vi "Init Filtered System Mappings Tab.vi"(8 "error in (no error)":errorcluster, 11 "Loop Data in":T1) -> (0 "error out":errorcluster)   [LabVIEW 2016, in "System Mapping Tool.lvlib"]
uses:
  System Mapping Tool.lvlib
  TypeDefs/Loop Data.ctl
  TypeDefs/UI Refs.ctl
  NationalInstruments.VeriStand.SystemDefinitionAPI
  NationalInstruments.VeriStand.SystemStorageUI
  <vilib>/Utility/miscctls.llb/LVRowAndColumnTypeDef.ctl
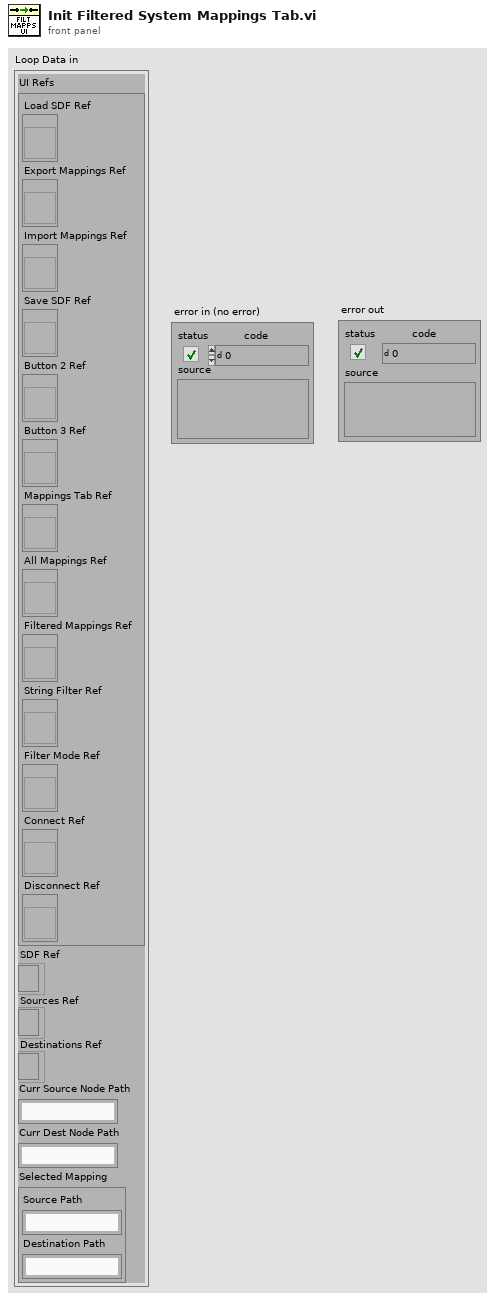
[diagram p1: front panel]
types:
  T1 = typedef "System Mapping Tool.lvlib/Loop Data.ctl" = cluster{"UI Refs":T2, "SDF Ref":refnum<k24>, "Sources Ref":refnum<k24>, "Destinations Ref":refnum<k24>, "Curr Source Node Path":string, "Curr Dest Node Path":string, "Selected Mapping":cluster{"Source Path":string, "Destination Path":string}}
  T2 = typedef "System Mapping Tool.lvlib/UI Refs.ctl" = cluster{"Load SDF Ref":refnum<vi>, "Export Mappings Ref":refnum<vi>, "Import Mappings Ref":refnum<vi>, "Save SDF Ref":refnum<vi>, "Button 2 Ref":refnum<vi>, "Button 3 Ref":refnum<vi>, "Mappings Tab Ref":refnum<vi>, "All Mappings Ref":refnum<vi>, "Filtered Mappings Ref":refnum<vi>, "String Filter Ref":refnum<vi>, "Filter Mode Ref":refnum<vi>, "Connect Ref":refnum<vi>, "Disconnect Ref":refnum<vi>}
  T3 = typedef "LVRowAndColumnTypeDef.ctl" = cluster{"Row":i32, "Column":i32}
  T4 = enum32{"All System Mappings", "Filtered Mappings by Node"}
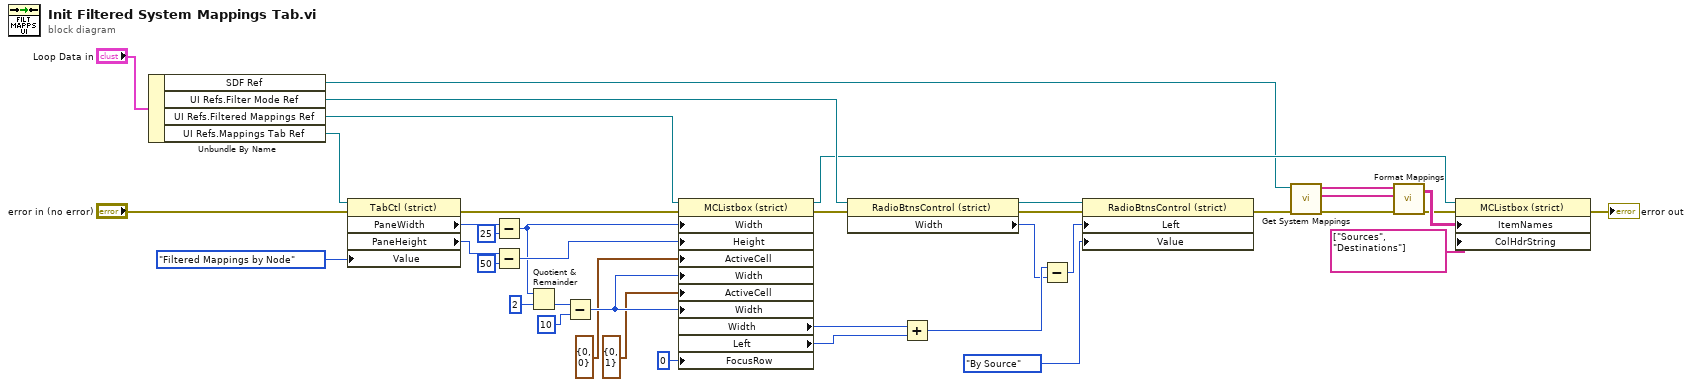
[diagram p0: block diagram]
diagram:
  n1 = Unbundle By Name("Loop Data in") -> ("SDF Ref"=w2:refnum<k24>, "UI Refs.Filter Mode Ref"=w18:refnum<vi>, "UI Refs.Filtered Mappings Ref"=w24:refnum<vi>, "UI Refs.Mappings Tab Ref"=w25:refnum<vi>)
  n2 = property class="TabCtl (strict)"(reference=w25, error in="error in (no error)", "Value"=T4."Filtered Mappings by Node") -> (error out=w38:errorcluster, "PaneWidth"=w31:u32, "PaneHeight"=w28:u32)  [unwired: 1 out]
  n3 = Subtract(x=w31, y=u32 25) -> (x-y=w26:u32)
  n4 = Subtract(x=w28, y=u32 50) -> (x-y=w27:u32)
  n5 = Quotient & Remainder(x=w26, y=u32 2) -> (floor(x/y)=w36:u32)  [unwired: 1 out]
  n6 = Subtract(x=w36, y=u32 10) -> (x-y=w34:u32)
  n7 = property class="MCListbox (strict)"(reference=w24, error in=w38, "Width"=w26, "Height"=w27, "ActiveCell"=T3 {"Row"=0, "Column"=0} ("Active Cell:Active Cell"), "Width"=w34, "ActiveCell"=T3 {"Row"=0, "Column"=1} ("Active Cell:Active Cell"), "Width"=w34, "FocusRow"=0 ("Focus Row")) -> (reference out=w8:refnum<vi>, error out=w16:errorcluster, "Width"=w20:u32, "Left"=w21:i32)
  n8 = property class="RadioBtnsControl (strict)"(reference=w18, error in=w16) -> (reference out=w17:refnum<vi>, error out=w19:errorcluster, "Width"=w14:u32)
  n9 = Add(x=w20, y=w21) -> (x+y=w15:u32)
  n10 = Subtract(x=w15, y=w14) -> (x-y=w13:u32)
  n11 = property class="RadioBtnsControl (strict)"(reference=w17, error in=w19, "Left"=w13, "Value"=enum32{"By Source", "By Destination"}."By Source") -> (error out=w10:errorcluster)  [unwired: 1 out]
  n12 = call "Get System Mappings.vi"("error in (no error)"=w10, "SDF Ref"=w2) -> ("error out"=w6:errorcluster, "Destinations"=w5:string[], "Sources"=w4:string[])  [unwired: 7 in]
  n13 = call "Format Mappings.vi"("Destinations"=w5, "Sources"=w4) -> ("Mappings"=w12:string[][])  [unwired: 3 in]
  n14 = property class="MCListbox (strict)"(reference=w8, error in=w6, "ItemNames"=w12, "ColHdrString"=string[] ["Sources", "Destinations"] ("Row Header Strings[]")) -> (error out=→"error out":errorcluster)  [unwired: 1 out]
